vi "Input DMA Engine.vi"(10 "Parameters":variant, 11 "Process":refnum<class "Process.lvclass">) -> ()   [LabVIEW 2016, in "FPGA Addon Engine.lvlib"]
uses:
  FPGA Addon Engine.lvlib
  <vilib>/NI/NIVS Inline Async API/_VS Inline Async API/Process/Process.lvclass
  Types/DMA Input References.ctl
  <vilib>/NI Veristand/Custom Device Waveform API/Multiple Waveforms Write (DBL)/Multiple Waveforms Write (DBL).lvclass
  Types/DMA Input Ref.ctl
  FPGA-Resource-Manager-APIs/Source/Shared/Types/DMA Settings.ctl
  FPGA-Resource-Manager-APIs/Source/Shared/Types/Delacing Scheme.ctl
  FPGA-Resource-Manager-APIs/Source/Shared/Types/DMA Acquisition Mode.ctl
  <vilib>/NI/NIVS Inline Async API/_VS Inline Async API/Process/Process.lvclass/Process.ctl
  <vilib>/Platform/TimedLoop/XDataNode/timing_clust.ctl
  <vilib>/Platform/TimedLoop/XDataNode/nitl_modes.ctl
  <vilib>/Platform/TimedLoop/XDataNode/wakeup.ctl
  <vilib>/NI/NIVS Inline Async API/_Data Access Engine/Access Type Classes/Write/Write.lvclass/Write.ctl
  <vilib>/NI/NIVS Inline Async API/_Data Access Engine/Data Access Engine/Methods/Write.Data.vi
  <vilib>/NI/NIVS Inline Async API/_VS Inline Async API/Process/Data Member Access/Read Data Access.vi
  <vilib>/NI/NIVS Inline Async API/_Data Access Engine/Access Type Classes/Write/Write.ProcessData.vi
  <vilib>/NI/NIVS Inline Async API/_VS Inline Async API/Error Handling Process/SubVIs/Error.ConvertArray.vi
  <vilib>/NI Veristand/Custom Device Waveform API/Multiple Waveforms Write (DBL)/NI VeriStand - Close Multiple Waveforms Write Session (DBL).vi
  <vilib>/FPGAPlugInAG/Dynamic/niLvFpga_Close_Dynamic.vi
  <vilib>/NI/NIVS Inline Async API/_Data Access Engine/Data Access Engine/Methods/Write.Lookup.vi
  <vilib>/rvi/interface/nirviCloseFPGA/nirviCloseFPGA.xnode
  <vilib>/Platform/TimedLoop/XDataNode/XDataNode.xnode
  <vilib>/NI/NIVS Inline Async API/_Data Access Engine/Data Access Engine/Data Access Engine.lvclass
  <vilib>/NI VeriStand/Custom Device Waveform API/NI_VS Custom Device Waveform API.lvlib
  <vilib>/NI VeriStand/Custom Device Tools/Custom Device Utility Library/Custom Device Utility Library.lvlib
  <vilib>/Platform/TimedLoop/XDataNode/XDNodeRunTimeDep.lvlib
  FPGA-Resource-Manager-APIs/Source/Shared/FPGA RM Shared API.lvlib
panel:
  out "error out":errorcluster
  in  "error in (no error)":errorcluster
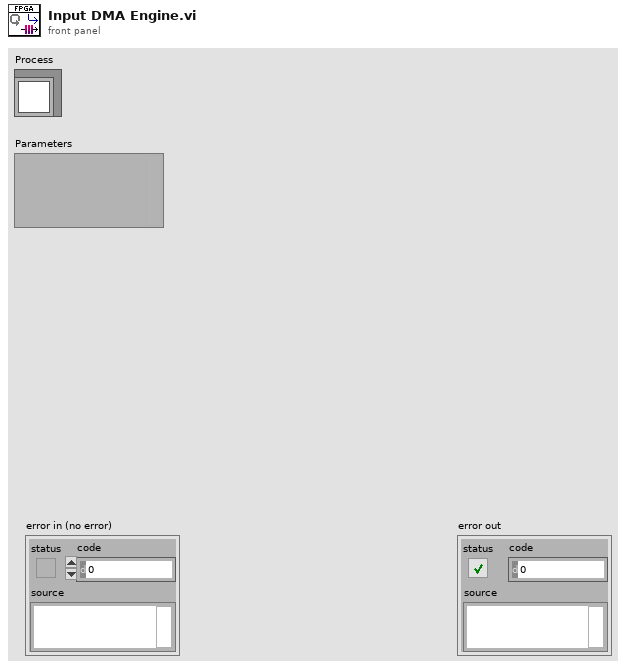
[diagram p1: front panel]
types:
  T1 = typedef "FPGA Addon Engine.lvlib/DMA Input References.ctl" = cluster{"Waveform Ref":refnum<class "Multiple Waveforms Write (DBL).lvclass">, "DMA Ref":T2, "Name":string, "DMA Settings":T3}
  T2 = typedef "FPGA Addon Engine.lvlib/DMA Input Ref.ctl" = refnum<k20>
  T3 = typedef "FPGA RM Shared API.lvlib/DMA Settings.ctl" = cluster{"Number of Channels":u8, "Delacing Scheme":T4, "Update Rate":u32, "dt":dbl, "Mode":T5, "Number of Samples":u32, "DMA Host Buffer":u32}
  T4 = typedef "FPGA RM Shared API.lvlib/Delacing Scheme.ctl" = enum8{"Interleaved"}
  T5 = typedef "FPGA RM Shared API.lvlib/DMA Acquisition Mode.ctl" = enum8{"Continuous", "Triggered Finite"}
  T6 = typedef "Data Access Engine.lvlib/Data Access Engine.lvclass/Write.DVR.ctl" = refnum<data-value>
  T7 = typedef "XDNodeRunTimeDep.lvlib/timing_clust.ctl" = cluster{"Expected End [f-1]":u64, "Actual End [f-1]":u64, "Finished Late? [f-1]":bool, "Expected End [i-1]":u64, "Actual End [i-1]":u64, "Finished Late? [i-1]":bool, "Expected Start [i]":u64, "Actual Start [i]":u64, "Expected Start [f]":u64, "Actual Start [f]":u64, "Source Name":string, "Structure Name":string, "Period":i64, "Deadline":i64, "Offset":i64, "Start":i64, "Priority":i32, "Timeout":i32, "Mode":T8, "Wakeup Reason":T9, "Error":errorcluster, "Source Type":string, "Secondary Source Type":string, "Global End Time":u64, "Global Start Time":u64, "Frame Duration":u64, "Iteration Duration":u64, "Assigned CPU":i32, "I/O Scan Engine Mode":u32}
  T8 = typedef "XDNodeRunTimeDep.lvlib/nitl_modes.ctl" = enum32{"No Change", "Process missed periods, maintain original phase", "Discard missed periods, maintain original phase", "Process missed periods, ignore original phase", "Discard missed periods, ignore original phase"}
  T9 = typedef "XDNodeRunTimeDep.lvlib/wakeup.ctl" = enum32{"Normal", "Aborted", "Asynchronous wakeup", "Timing source error", "Timed loop error", "Timeout"}
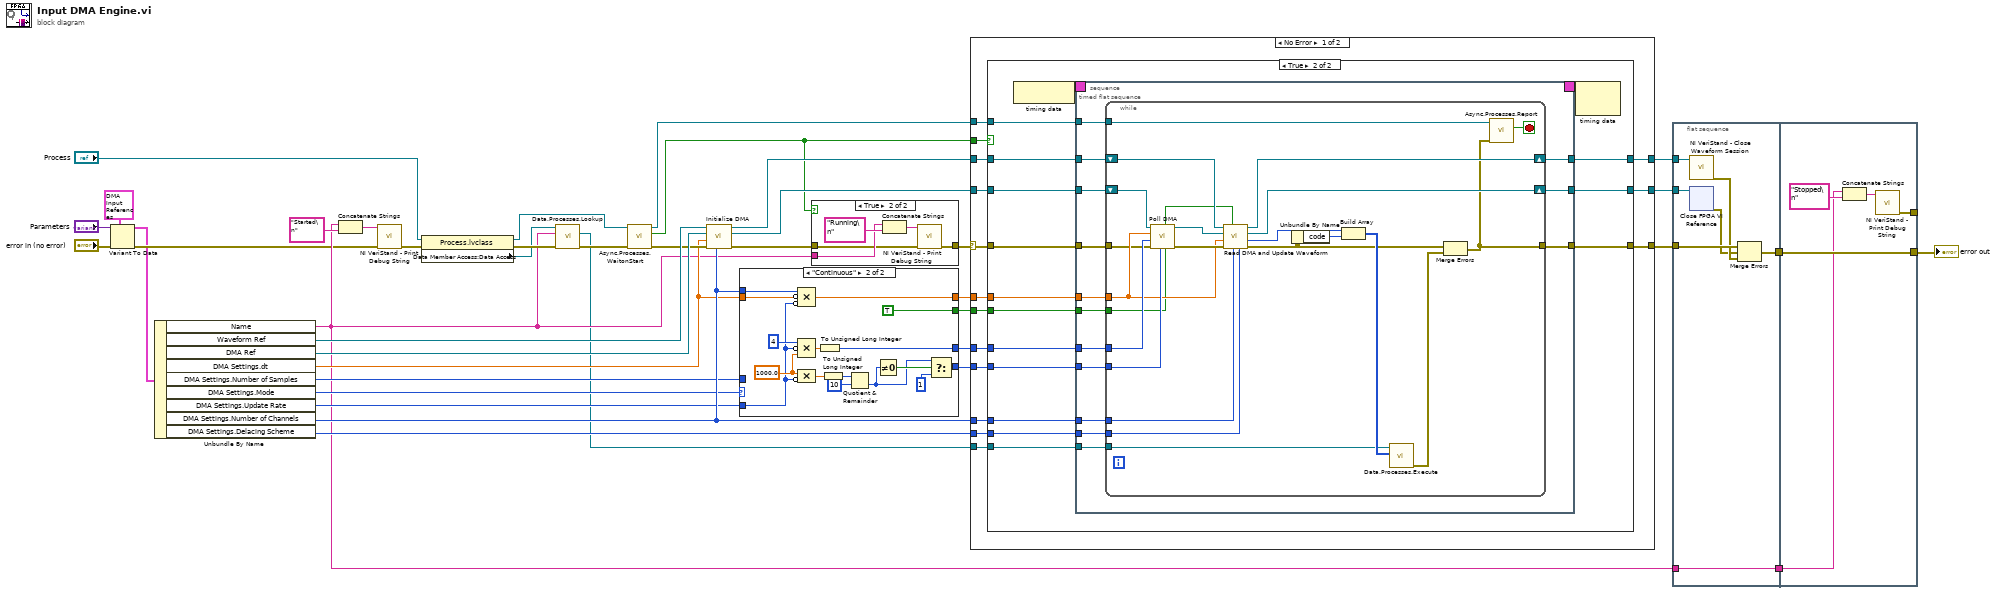
[diagram p0: block diagram]
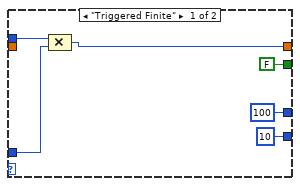
[diagram p2: hidden frame]
diagram:
  n1 = Variant To Data(error in="error in (no error)", type=T1 {"Waveform Ref"=refnum, "DMA Ref"=refnum, "Name"="", "DMA Settings"={"Number of Channels"=0, "Delacing Scheme"=enum."Interleaved", "Update Rate"=0, "dt"=1000.0, "Mode"=enum."Continuous", "Number of Samples"=10000, "DMA Host Buffer"=5}} ("Parameters"), Variant="Parameters") -> (data=w2:T1, error out=w4:errorcluster)
  n2 = Unbundle By Name(w2) -> ("Name"=w7:string, "Waveform Ref"=w40:refnum<class "Multiple Waveforms Write (DBL).lvclass">, "DMA Ref"=w29:T2, "DMA Settings.dt"=w19:dbl, "DMA Settings.Number of Samples"=w14:u32, "DMA Settings.Mode"=w15:T5, "DMA Settings.Update Rate"=w18:u32, "DMA Settings.Number of Channels"=w20:u8, "DMA Settings.Delacing Scheme"=w30:T4)
  n3 = Concatenate Strings(w7, "Started\n" ("string")) -> (w34:string)
  n4 = call <vilib>:"NI VeriStand - Print Debug String.vi"("error in (no error)"=w4, "Message"=w34) -> ("error out"=w11:errorcluster)  [unwired: 9 in]
  n5 = property class="Process.lvclass"(reference="Process", error in=w11) -> (reference out=w12:refnum<class "Process.lvclass">, error out=w10:errorcluster, "Data Member Access:Data Access"=w8:refnum<class "Data Access Engine.lvclass">)
  n6 = call-poly <vilib>:"Data.Processes.Lookup.vi"("error in (no error)"=w10, "Name"=w7, "Data Access API in"=w8) -> ("error out"=w9:errorcluster, "Ref"=w6:T6)  [unwired: 5 in, 2 out]
  n7 = call <vilib>:"Async.Processes.WaitonStart.vi"("error in (no error)"=w9, "Process"=w12) -> ("error out"=w26:errorcluster, "Execute"=w27:bool, "Process out"=w5:refnum<class "Process.lvclass">)  [unwired: 7 in]
  n8 = call "Initialize DMA.vi"("Number of Channels"=w20, "error in (no error)"=w26, "dt"=w19, "DMA Ref"=w29, "Multiple Waveforms Write (DBL) in"=w40) -> ("error out"=w25:errorcluster, "DMA Ref"=w38:T2, "Multiple Waveforms Write (DBL) out"=w39:refnum<class "Multiple Waveforms Write (DBL).lvclass">)  [unwired: 4 in]
  n9 = case shown="\"Continuous\"" w15 {
    tunnel: [u32 10 ("f") w55] -> w22
    tunnel: [u32 100 w52] -> w21
    tunnel: w20 -> [w46 w51]
    tunnel: w19 -> [_ w50]
    tunnel: w18 -> [_ w49]
    tunnel: [w44 w48] -> w17
    tunnel: [FALSE TRUE] -> w16
    tunnel: w14 -> [w45 _]
    frame "Triggered Finite" {
      n10 = Compound Arithmetic op=MULTIPLY(w46, w45) -> (w44:u32)
    }
    frame "Continuous" {
      w53 = 1000.0 ("y")
      n11 = Compound Arithmetic op=MULTIPLY(w51, invert w50, invert w49) -> (w48:dbl)
      n12 = Compound Arithmetic op=MULTIPLY(u32 4 ("value"), invert w49, w53) -> (w54:dbl)
      n13 = Compound Arithmetic op=MULTIPLY(w53, invert w49) -> (w57:dbl)
      n14 = To Unsigned Long Integer(number=w54) -> (unsigned 32bit integer=w52:u32)
      n15 = To Unsigned Long Integer(number=w57) -> (unsigned 32bit integer=w58:u32)
      n16 = Quotient & Remainder(x=w58, y=u32 10) -> (floor(x/y)=w56:u32)  [unwired: 1 out]
      n17 = Not Equal To 0?(x=w56) -> (x != 0?=w61:bool)
      n18 = Select(t=w56, s=w61, f=u32 1) -> (s? t:f=w55:u32)
    }
  }
  n19 = case shown="True" w27 {
    tunnel: w7 -> [_ w66]
    tunnel: w25 -> [w63 w65]
    tunnel: [w63 w64] -> w24
    frame False {
    }
    frame True {
      n20 = Concatenate Strings(w66, "Running\n" ("string")) -> (w68:string)
      n21 = call <vilib>:"NI VeriStand - Print Debug String.vi"("error in (no error)"=w65, "Message"=w68) -> ("error out"=w64:errorcluster)  [unwired: 9 in]
    }
  }
  n22 = case shown="No Error" w24 {
    selector: w24 -> [w75 w160]
    tunnel: w39 -> [w83 w159]
    tunnel: w38 -> [w82 w158]
    tunnel: w17 -> [w81 _]
    tunnel: w20 -> [w80 _]
    tunnel: [w79 w159] -> w37
    tunnel: [w78 w160] -> w36
    tunnel: w21 -> [w77 _]
    tunnel: w5 -> [w76 _]
    tunnel: w27 -> [w74 _]
    tunnel: w22 -> [w73 _]
    tunnel: [w72 w158] -> w32
    tunnel: w30 -> [w71 _]
    tunnel: w6 -> [w70 _]
    tunnel: w16 -> [w69 _]
    frame No Error {
      n23 = case shown="True" w74 {
        tunnel: w83 -> [w86 w102]
        tunnel: w82 -> [w84 w101]
        tunnel: w81 -> [_ w100]
        tunnel: w80 -> [_ w99]
        tunnel: [w86 w98] -> w79
        tunnel: [w85 w91] -> w78
        tunnel: w77 -> [_ w97]
        tunnel: w76 -> [_ w96]
        tunnel: w75 -> [w85 w90]
        tunnel: w73 -> [_ w95]
        tunnel: [w84 w94] -> w72
        tunnel: w71 -> [_ w93]
        tunnel: w70 -> [_ w92]
        tunnel: w69 -> [_ w89]
        frame False {
        }
        frame True {
          n24 = node-c288() -> (w88:T7)
          n25 = timed-sequence {
            timing: w88 -> [_]
            timing-out: [_] -> w87
            tunnel: w102 -> [w116]
            tunnel: w101 -> [w115]
            tunnel: w100 -> [w114]
            tunnel: w99 -> [w113]
            tunnel: [w112] -> w98
            tunnel: w97 -> [w111]
            tunnel: w96 -> [w110]
            tunnel: w95 -> [w109]
            tunnel: [w108] -> w94
            tunnel: w93 -> [w107]
            tunnel: w92 -> [w106]
            tunnel: [w105] -> w91
            tunnel: w90 -> [w104]
            tunnel: w89 -> [w103]
            n26 = timed-flat-sequence {
              tunnel: w116 -> [w130]
              tunnel: w115 -> [w129]
              tunnel: w114 -> [w128]
              tunnel: w113 -> [w127]
              tunnel: [w126] -> w112
              tunnel: w111 -> [w125]
              tunnel: w110 -> [w124]
              tunnel: w109 -> [w123]
              tunnel: [w122] -> w108
              tunnel: w107 -> [w121]
              tunnel: w106 -> [w120]
              tunnel: [w119] -> w105
              tunnel: w104 -> [w118]
              tunnel: w103 -> [w117]
              n27 = while {
                tunnel: w125 -> [w151]
                tunnel: w128 -> [w139]
                tunnel: w127 -> [w138]
                tunnel: w124 -> [w149]
                tunnel: w123 -> [w147]
                tunnel: w121 -> [w137]
                tunnel: w120 -> [w144]
                shift-right: [w141] -> w122
                shift-left: w129 -> [w152]
                shift-right: [w150] -> w126
                shift-left: w130 -> [w153]
                tunnel: [w135] -> w119
                tunnel: w118 -> [w134]
                tunnel: w117 -> [w132]
                stop <- w131 stop-if-true
                n28 = call "Poll DMA.vi"("Timeout is Error?"=w132, "Wait (ms)"=w147, "error in (no error)"=w134, "Timeout (ms)"=w151, "Total Samples to Read"=w139, "DMA Ref"=w152) -> ("error out"=w148:errorcluster, "DMA Ref"=w140:T2, "Timeout?"=w133:bool)  [unwired: 3 in]
                n29 = call "Read DMA and Update Waveform.vi"("Delacing Scheme"=w137, "Number of Channels"=w138, "Timeout?"=w133, "error in (no error)"=w148, "Total Samples"=w139, "DMA Ref"=w140, "Multiple Waveforms Write (DBL) in"=w153) -> ("error out"=w136:errorcluster, "Elements Remaining"=w142:u32, "FPGA VI Reference Out"=w141:T2, "Multiple Waveforms Write (DBL) out"=w150:refnum<class "Multiple Waveforms Write (DBL).lvclass">)  [unwired: 1 in]
                n30 = Unbundle By Name(w136) -> ("code"=w146:i32)
                n31 = Build Array(w142, w146) -> (w145:u32[])
                n32 = call-poly <vilib>:"Data.Processes.Execute.vi"("Values"=w145, "Ref"=w144) -> ("error out"=w143:errorcluster)  [unwired: 9 in]
                n33 = Merge Errors(w136, w143) -> (w135:errorcluster)
                n34 = call <vilib>:"Async.Processes.Report.vi"("Error"=w135, "Process in"=w149) -> ("Stop"=w131:bool)  [unwired: 8 in, 1 out]
              }
            }
          }
          n35 = node-c288(w87) -> ()  [unwired: 1 out]
        }
      }
    }
    frame Error {
    }
  }
  n36 = flat-sequence {
    tunnel: w37 -> [w167]
    tunnel: w36 -> [w166]
    tunnel: w32 -> [w163]
    tunnel: [w164] -> w28
    tunnel: [w161] -> w23
    tunnel: w7 -> [w161]
    tunnel: [w172] -> w31
    tunnel: w28 -> [w172]
    tunnel: w23 -> [w169]
    tunnel: [w168] -> _
    frame #0 {
      n37 = call-poly <vilib>:"NI VeriStand - Close Waveform Session.vi"("Multiple Waveforms Write Session (DBL)"=w167) -> ("error out"=w165:errorcluster)  [unwired: 10 in]
      n38 = xnode "Close FPGA VI Reference"("FPGA VI Reference In"=w163) -> ("error out"=w162:errorcluster)  [unwired: 1 in]
      n39 = Merge Errors(w166, w162, w165) -> (w164:errorcluster)
    }
    frame #1 {
      n40 = Concatenate Strings(w169, "Stopped\n" ("string")) -> (w170:string)
      n41 = call <vilib>:"NI VeriStand - Print Debug String.vi"("Message"=w170) -> ("error out"=w168:errorcluster)  [unwired: 10 in]
    }
  }
  "error out" <- w31
